vi "Helium Pre Pulse Mag (Read).vi"(6 "ISOBUS address":T3=-1 caption="ISOBUS address (-1)", 8 "error in":errorcluster, 11 "Mercury Reference In":T4) -> (0 "error out":errorcluster, 1 "Unit":T1, 2 "Magnitude":dbl caption="Pre-pulse Magnitude (mA)", 3 "Mercury Reference Out":T4, 4 "Valid?":T2)   [LabVIEW 2019, in "Mercury iXX.lvlib" / "Level Meter.lvlib"]
doc: "Read the currently configured pre-pulse magnitude."
uses:
  Level Meter.lvlib
  Controls/Mercury Reference.ctl
  CryoTUM_20210311/sub_vi-s/Equipment/Mercury iXX/Public/Controls/Comms Transport Layer.ctl
  Private/Controls/Query Dynamic Reference.ctl
  Controls/ISOBus Address.ctl
  Controls/Is Valid LED.ctl
  Controls/Unit String.ctl
  Private/Controls/Command Verbs.ctl
  mercury/Mercury iXX.lvlib
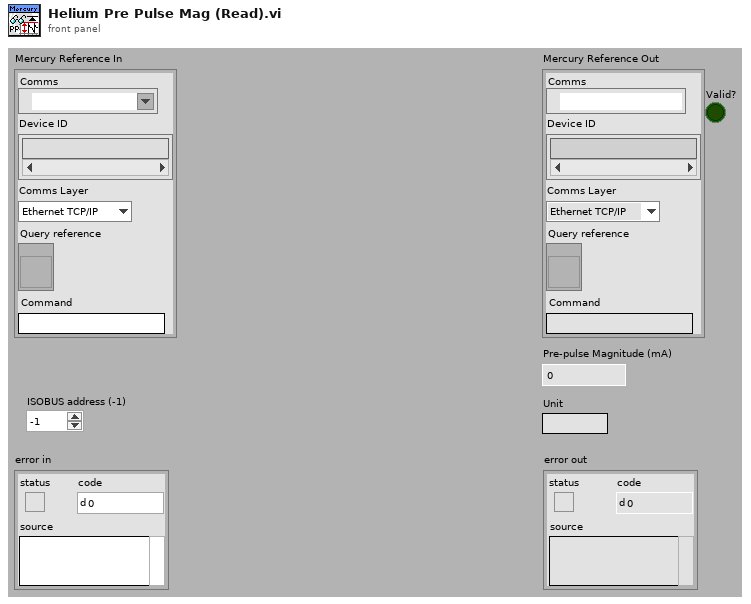
[diagram p1: front panel]
types:
  T1 = typedef "Mercury iXX.lvlib/Unit String.ctl" = string
  T2 = typedef "Mercury iXX.lvlib/Is Valid LED.ctl" = bool
  T3 = typedef "Mercury iXX.lvlib/ISOBus Address.ctl" = i32
  T4 = typedef "Mercury iXX.lvlib/Mercury Reference.ctl" = cluster{"Comms":refnum<visa-resource-name>, "Device ID":string[], "Comms Layer":T5, "Command":string, "Query reference":T6}
  T5 = typedef "Mercury iXX.lvlib/Comms Transport Layer.ctl" = enum16{"Ethernet TCP/IP", "USB", "ISOBus - RS-232", "GPIB"}
  T6 = typedef "Mercury iXX.lvlib/Query Dynamic Reference.ctl" = refnum<vi>
  T7 = typedef "Mercury iXX.lvlib/Command Verbs.ctl" = string
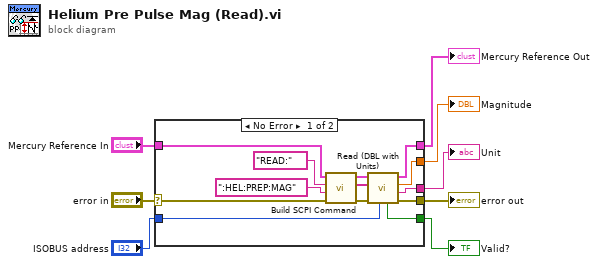
[diagram p0: block diagram]
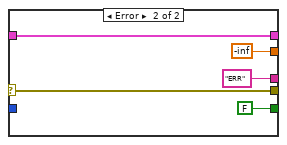
[diagram p2: hidden frame]
diagram:
  n1 = case shown="No Error" "error in" {
    selector: "error in" -> [w20 w26]
    tunnel: "Mercury Reference In" -> [w21 w25]
    tunnel: [w14 w25] -> w5
    tunnel: [w9 w26] -> w4
    tunnel: "ISOBUS address" -> [w11 _]
    tunnel: [w12 T2 FALSE ("Valid?")] -> w3
    tunnel: [w13 -inf] -> w2
    tunnel: [w15 T1 "ERR" ("Unit")] -> w1
    frame No Error {
      n2 = call "Build SCPI Command.vi"("error in"=w20, "Noun(s)"=":HEL:PREP:MAG" ("Command"), "Verb"=T7 "READ:", "Mercury Reference In"=w21) -> ("error out"=w17:errorcluster, "SCPI Message(s)"=w10:string[], "Mercury Reference Out"=w16:T4)  [unwired: 5 out]
      n3 = call "Read (DBL with Units).vi"("ISOBUS address"=w11, "error in"=w17, "SCPI Message(s)"=w10, "Mercury Reference In"=w16) -> ("error out"=w9:errorcluster, "Unit"=w15:T1, "Data (Dbl)"=w13:dbl, "Mercury Reference Out"=w14:T4, "Valid?"=w12:T2)  [unwired: 3 out]
    }
    frame Error {
    }
  }
  "Mercury Reference Out" <- w5
  "error out" <- w4
  "Valid?" <- w3
  "Unit" <- w1
  "Magnitude" <- w2
